vi "Unreserve Session(s).vi"   [LabVIEW 2020, in "NIDCPowerSourceDCVoltage.lvlib"]
uses:
  NIDCPowerSourceDCVoltage.lvlib
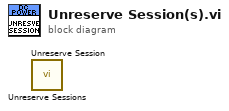
[diagram p0: block diagram]
diagram:
  n1 = call "Unreserve Sessions.vi"() -> ()  [unwired: 11 in, 1 out]
  n2 = call "Unreserve Session.vi"() -> ()  [unwired: 11 in, 1 out]
